vi "cRIO_FPGA_COMMUNICATION Zähler_Konfigurieren.vi"(3 "Zählerconfiguration":T2, 4 "Zähler":enum16{"Zähler 1", "Zähler 2", "Zähler 3"}(ring), 5 "Station Index":T1) -> ()   [LabVIEW 2013, in "cRIO_FPGA_COMMUNICATION.lvlib"]
uses:
  cRIO_FPGA_COMMUNICATION.lvlib
  TYPES/TYPE Station Index.ctl
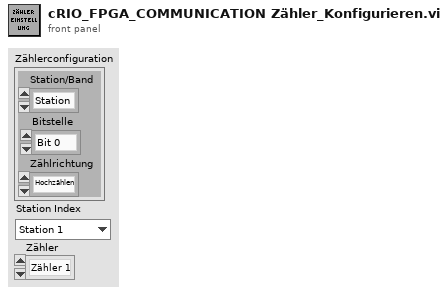
[diagram p1: front panel]
types:
  T1 = typedef "cRIO_FPGA_COMMUNICATION.lvlib/TYPE Station Index.ctl" = enum16{"Station 1", "Station 2", "Station 3", "Station 4", "Station 5", "Station 6", "Station 7", "Station 8", "Station 9", "Station 10", "Station 11", "Station 12", "Station 13", "Station 14", "Station 15", "Station 16", "Station 17", "Station 18", "Station 19", "Station 20"}
  T2 = cluster{"Station/Band":enum16{"Station", "Band"}, "Bitstelle":enum16{"Bit 0", "Bit 1", "Bit 2", "Bit 3", "Bit 4", "Bit 5", "Bit 6", "Bit 7"}, "Zählrichtung":enum16{"Hochzählen", "Runterzählen"}}
  T3 = enum16{"Init", "set Counter", "get Counter", "reset Counter", "configure Counter"}
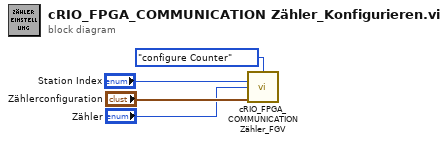
[diagram p0: block diagram]
diagram:
  n1 = call "cRIO_FPGA_COMMUNICATION Zähler_FGV.vi"("Set/Get/Configure"=T3."configure Counter", "Station Index"="Station Index", "Zähler"="Zähler", "Zählerconfiguration"="Zählerconfiguration") -> ()  [unwired: 10 in, 2 out]
